vi "Delta_RH_Auto_T-waiting_simple.vi"() -> ()   [LabVIEW 2012]
uses:
  <vilib>/ptbypt/NI_PtbyPt.lvlib
panel:
  in  "T-ramp off":bool
  in  "Set He3 Temp 2":bool
  in  "Main sorb T control":bool
  in  "Wait [min]":i32
  in  "1:Main   2:Mini":dbl=1.0
  in  "LakeShore335":refnum<visa-resource-name>="COM4"
  in  "Set He3 Temp":bool
  in  "Set temp [K]":dbl=1.0
  in  "rate [K/min]":dbl=5.0
  out "Main-sorb[K]":dbl=11.567
  out "Mini sorb [K]":dbl=4.35
  in  "Temp control off":bool=TRUE
  out "temp [K]":dbl=10.729
  out "Waiting T-stability":bool caption="stabilizing"
  in  "Set Initial Field":bool
  in  "Field [T]":dbl
  in  "Period [s]":dbl=0.5 caption="Delay Time (s)"
  in  "Measure R-T":bool
  in  "Save R-T":bool
  out "R-T":cluster{"X":dbl[], "Y":dbl[]}[](graph) caption="XY Graph"
  out "Rate [K/min]":dbl=0.0015950964745404326 format="%#_6f"
  in  "Reset":bool
  in  "Stop":bool
  in  "Pause off":bool
  in  "Compliance [V]":dbl=0.5 format="%#_6f"
  out "R-H":cluster{"X":dbl[], "Y":dbl[]}[](graph)=[{"X"=[0.00063, 0.00151, 0.00233, 0.003, 0.00367, 0.00427], "Y"=[11.5344858, 11.4030008, 11.9276791, 11.5452003, 11.5064993, 11.6247473]}] caption="XY Graph"
  in  "Reset":bool
  in  "Folder":path=path "C:/User Data/Angelo/Cr-doped_NbS2/Device_Nov_2018" caption="Filename"
  out "Filename Out":path=path "C:/User Data/Angelo/Cr-doped_NbS2/Device_Nov_2018/RH-junction5-1uA_0.30K"
  in  "File name":string="RH-junction5-1uA"
  out "VTI [K]":dbl=2.07338
  out "VTI [K]":dbl=2.07412
  out "Sample Temp [K]":dbl=0.70413
  out "Magnetic Field [T]":dbl=0.00483
  out "Delta reading [Ohm]":dbl=11.5541515
  out "Delta Reading [Ohm]":dbl=11.9426813
  out "Sample Temp [K]":dbl=0.70382
  in  "Abort Delta":bool
  in  "Arm Delta":bool
  in  "DELAY [sec]":dbl=0.002 format="%#_6e"
  in  "I-HIGH [A]":dbl=1e-06 format="%#_6e"
  in  "Measure R-H":bool
  in  "Rate [K/min]":dbl=0.5
  in  "Set Temp [K]":dbl=1.0
  in  "Set Temperature":bool
  out "Magnetic Field [T]":dbl
  in  "Rate [T/min]":dbl=0.1
  in  "Set Field [T]":dbl=-0.6
  in  "Set Field":bool
  in  "Keithley":refnum<visa-resource-name>="GPIB0::20::INSTR"
  in  "Skip":bool
  in  "Wait T-stable [min]":i32=20
  in  "period (s)":dbl=0.5 min=0.0 max=1111.0 step=0.1
  in  "stop 2":bool caption="Pause"
  in  "Wait field stable [sec]":dbl=20.0
  in  "Magnet Power supply":refnum<visa-resource-name>="COM6"
  in  "Set Field [T]   Rate [T/min]":dbl[][](array[numeric])=[[0.1, 0.04], [0.6, 0.1], [0.1, 0.1], [0.0, 0.04]]
  in  "Set Temp [K]  Rate [K/min]":dbl[][](array[numeric])=[[0.3, 0.2]]
  in  "LakeShore350":refnum<visa-resource-name>="COM5"
  out "error out 3":errorcluster={"status"=FALSE, "code"=1073676294, "source"="VISA Read in Delta_RH_Auto_T-waiting_simple.vi"}
  out "error out 2":errorcluster={"status"=TRUE, "code"=-1073807339, "source"="VISA Read in Delta_RH_Auto_T-waiting_simple.vi"}
  out "error out":errorcluster={"status"=FALSE, "code"=1073676294, "source"="VISA Read in Delta_RH_Auto_T-waiting_simple.vi"}
  # "Manual control"
  # "R-H Auto Measurement"
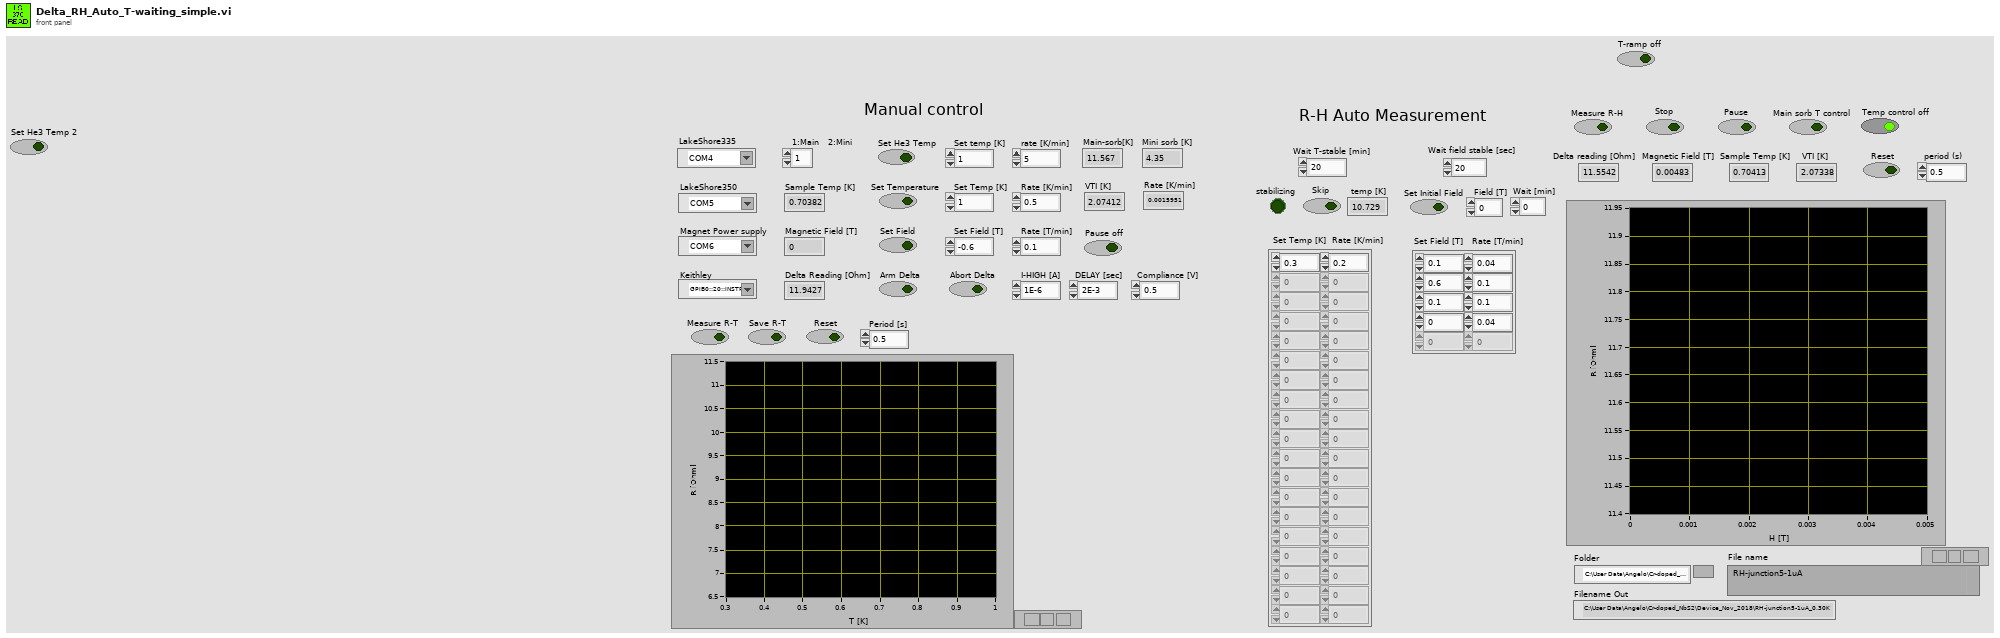
[diagram p1: front panel]
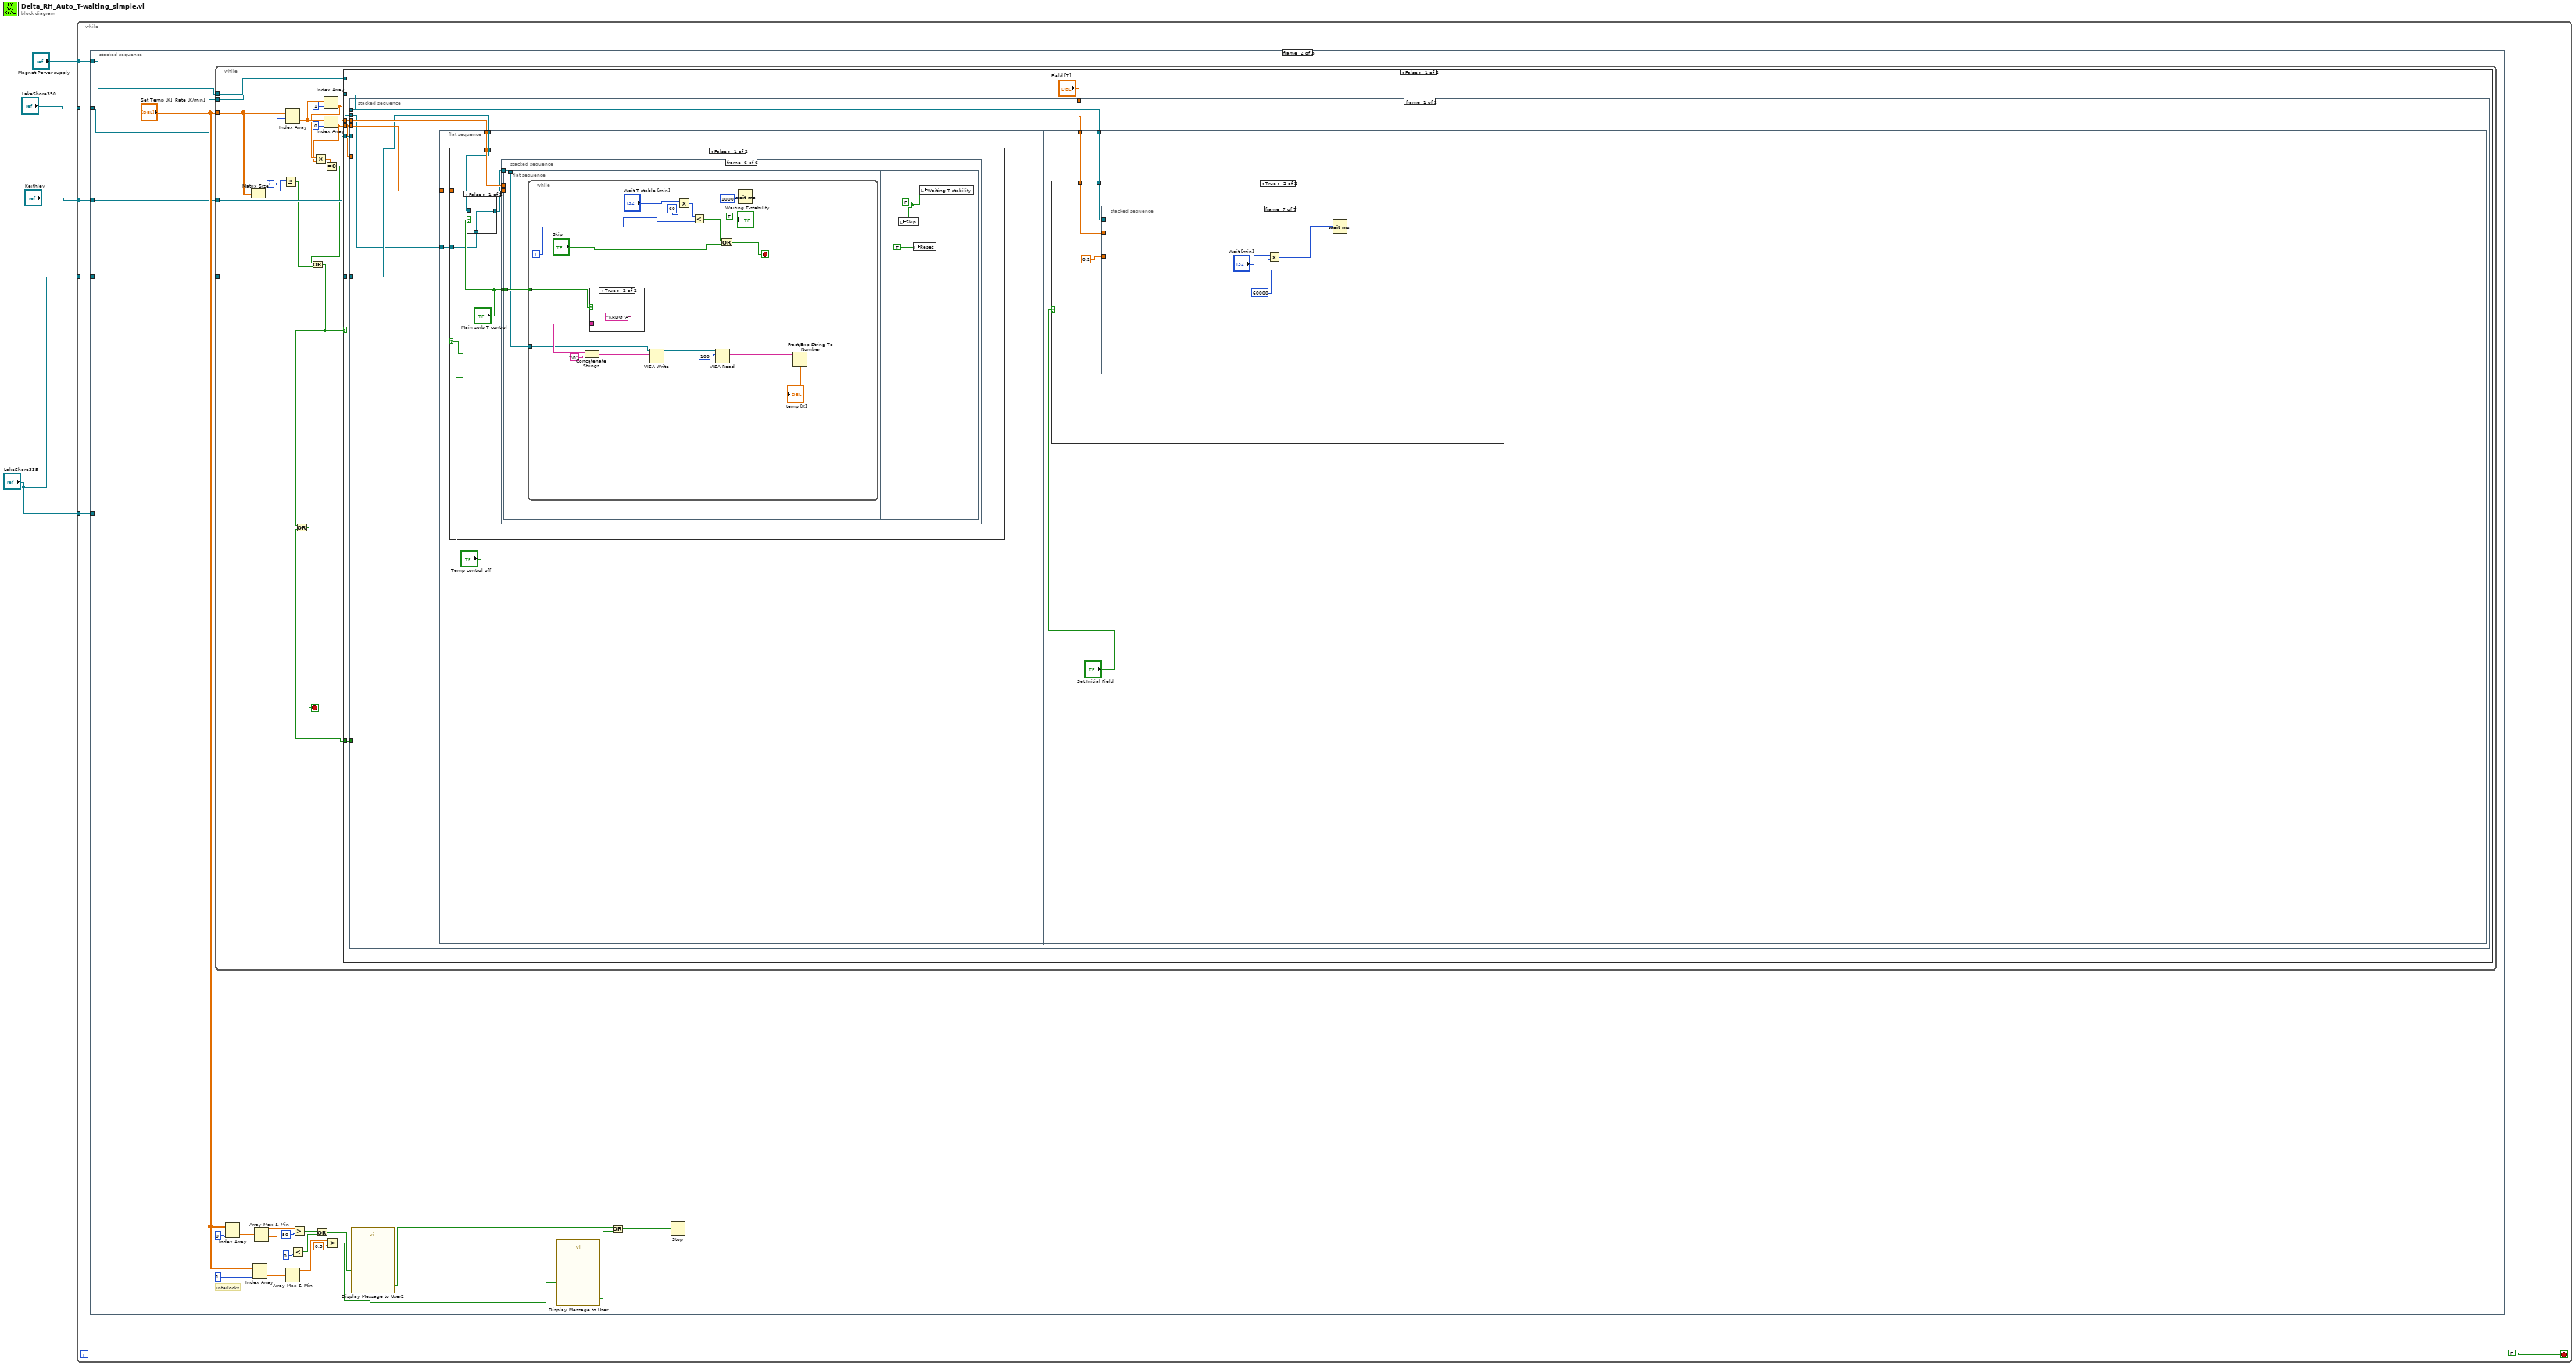
[diagram p0: block diagram]
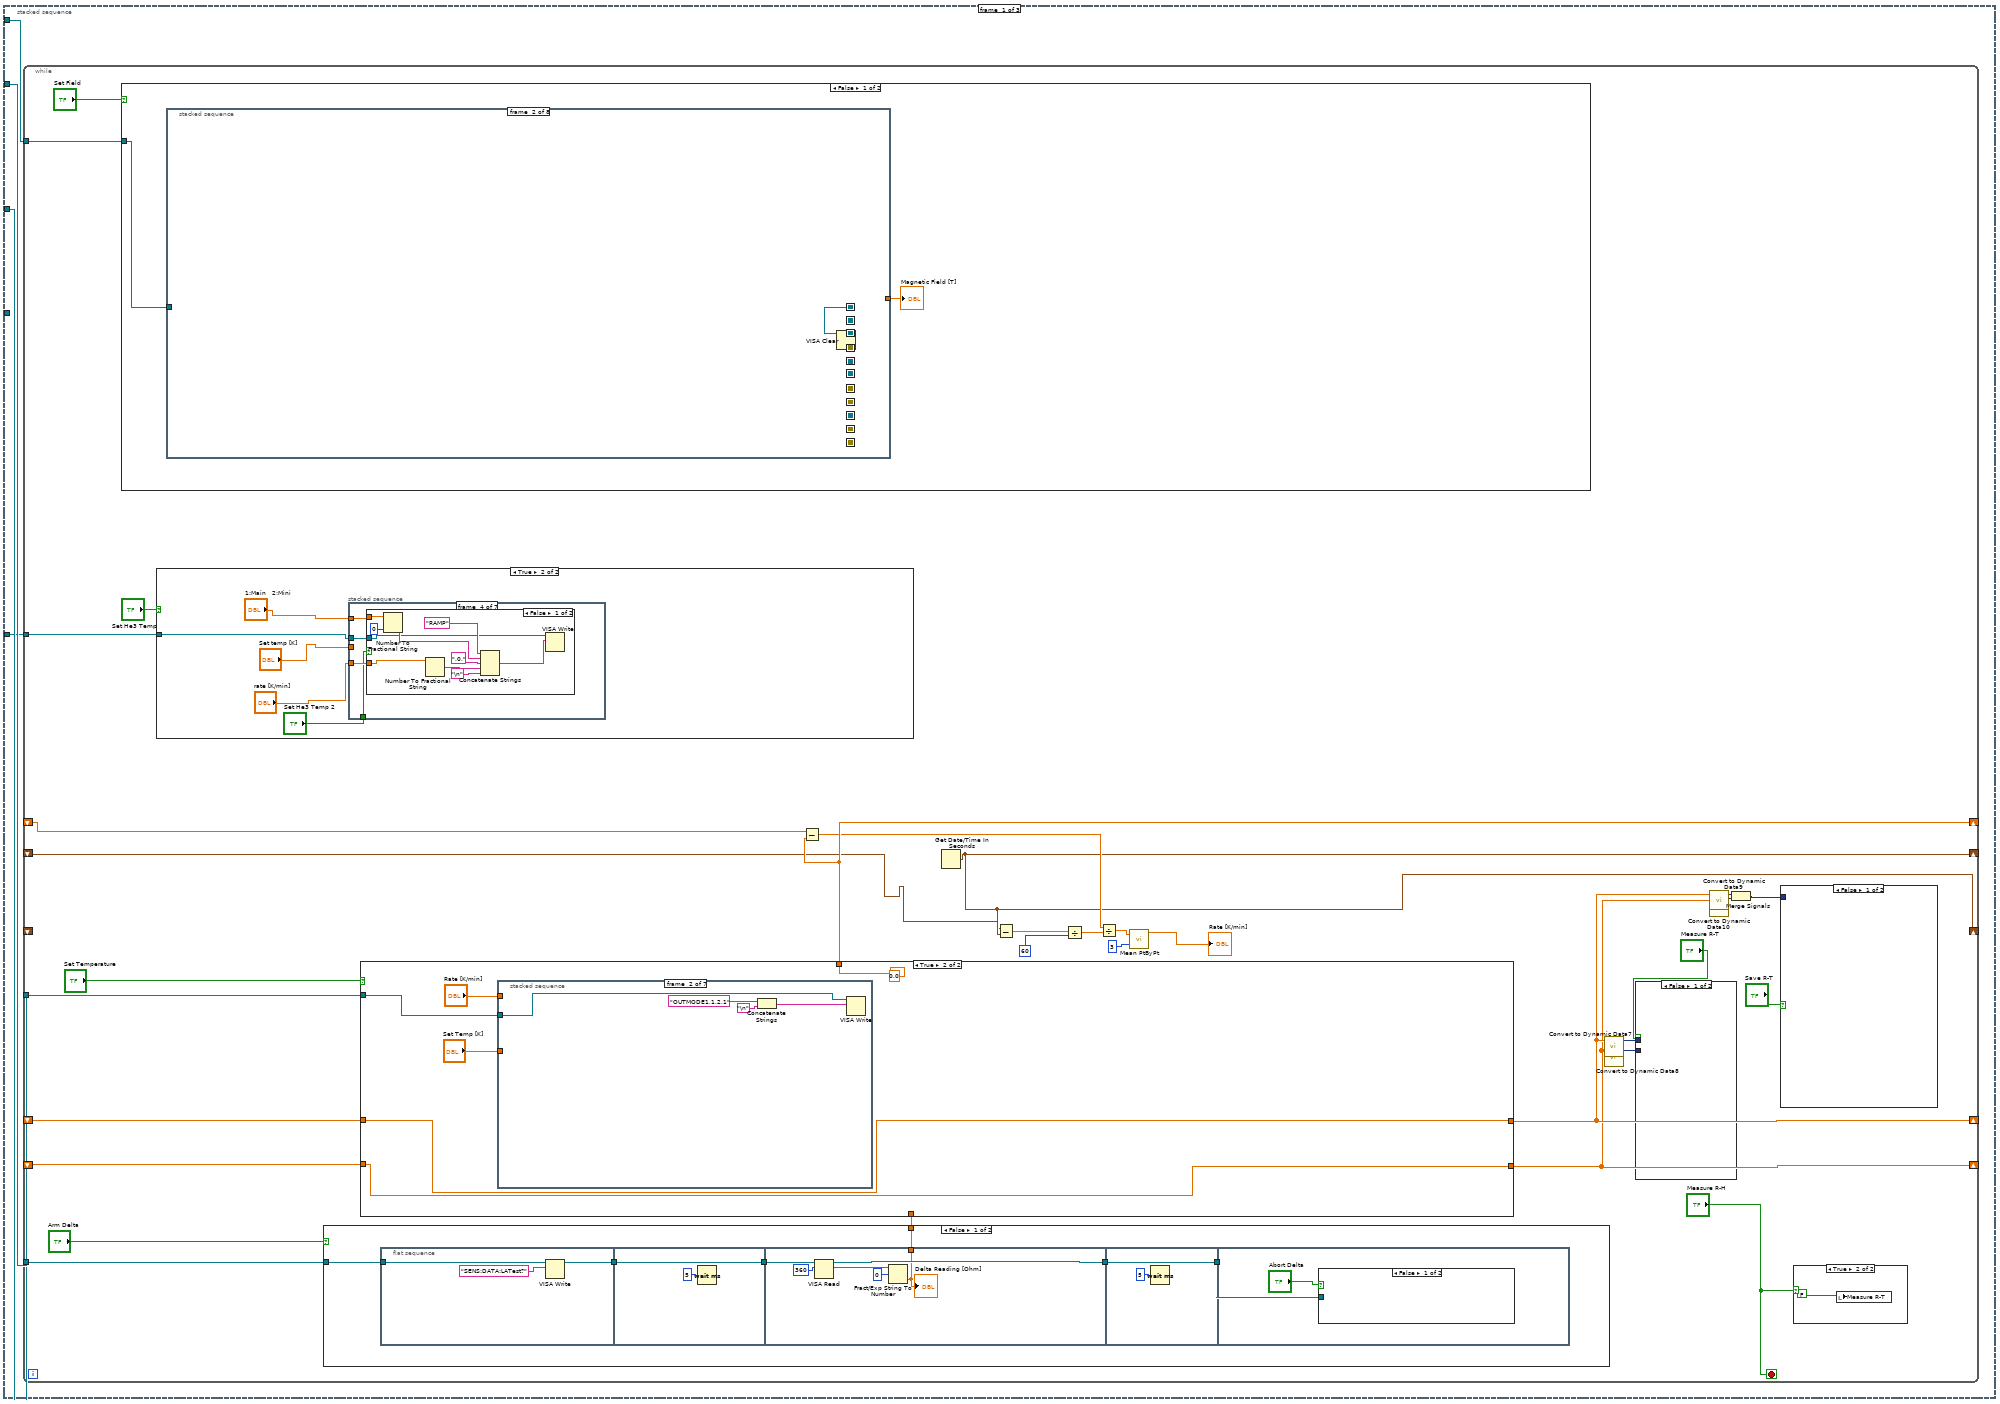
[diagram p2: hidden frame]
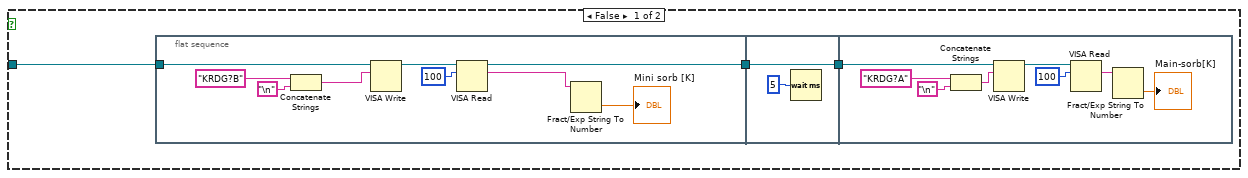
[diagram p3: hidden frame]
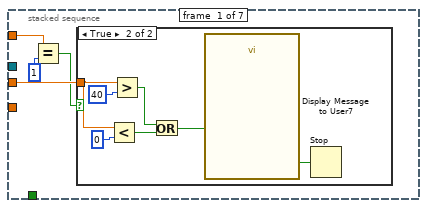
[diagram p4: hidden frame]
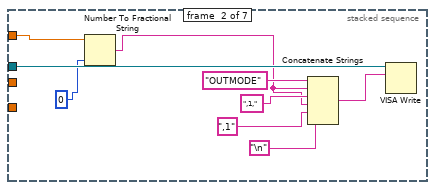
[diagram p6: hidden frame]
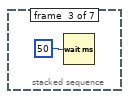
[diagram p7: hidden frame]
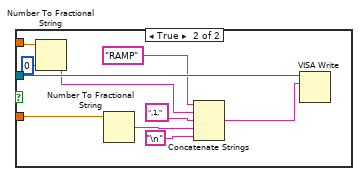
[diagram p8: hidden frame]
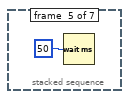
[diagram p9: hidden frame]
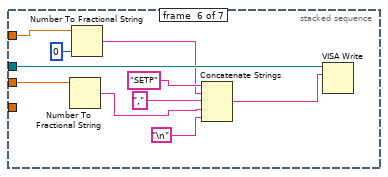
[diagram p10: hidden frame]
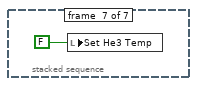
[diagram p11: hidden frame]
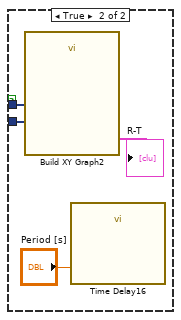
[diagram p13: hidden frame]
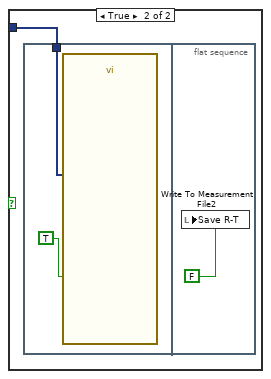
[diagram p14: hidden frame]
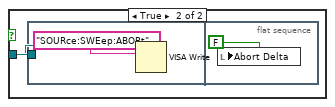
[diagram p15: hidden frame]
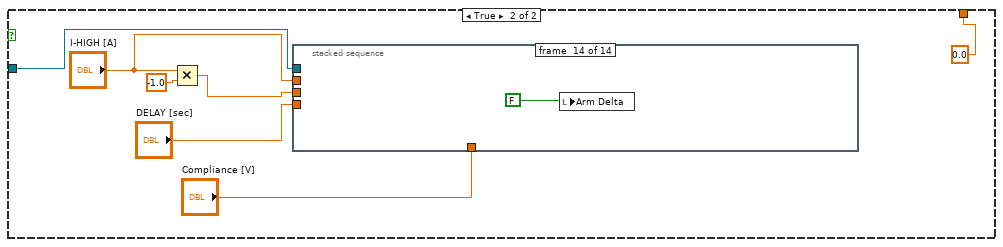
[diagram p16: hidden frame]
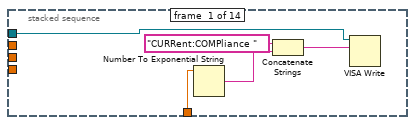
[diagram p17: hidden frame]
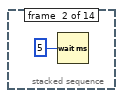
[diagram p18: hidden frame]
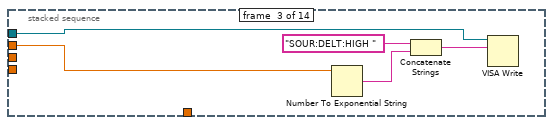
[diagram p19: hidden frame]
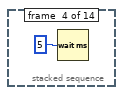
[diagram p20: hidden frame]
diagram:
  n1 = while {
    tunnel: "LakeShore350" -> [w10]
    tunnel: "Magnet Power supply" -> [w9]
    tunnel: "Keithley" -> [w8]
    tunnel: "LakeShore335" -> [w6]
    tunnel: "LakeShore335" -> [w5]
    stop <- FALSE stop-if-true
    n2 = stacked-sequence {
      tunnel: w10 -> [w13 w448 _]
      tunnel: w9 -> [w14 w447 w930]
      tunnel: w8 -> [w12 w446 _]
      tunnel: w6 -> [_ w444 _]
      tunnel: w5 -> [w11 _ _]
      frame #0 {
        n3 = while {
          tunnel: w14 -> [w41]
          tunnel: w13 -> [w44]
          tunnel: w12 -> [w43]
          shift-right: [w29] -> _
          shift-left: _ -> [w24]
          shift-right: [w27] -> _
          shift-left: _ -> [w39]
          shift-right: [w21] -> _
          shift-left: _ -> [_]
          shift-right: [w37] -> _
          shift-left: _ -> [w38]
          shift-right: [w21] -> _
          shift-left: _ -> [w20]
          tunnel: w11 -> [w15]
          stop <- "Measure R-H" stop-if-true
          n4 = case shown="False" "Set Field" {
            tunnel: w41 -> [w279 w349]
            frame False {
              n5 = stacked-sequence {
                seq-local: [w280 _ _ _ _ _ _ _] -> [_ w283 _ _ _ _ _ _]
                seq-local: [_ w281 _ _ _ _ _ _] -> [_ _ w287 _ _ _ _ _]
                seq-local: [_ w282 _ _ _ _ _ _] -> [_ _ w284 _ _ _ _ _]
                seq-local: [_ _ w286 _ _ _ _ _] -> [_ _ _ w327 _ _ _ _]
                seq-local: [_ _ w285 _ _ _ _ _] -> [_ _ _ w326 _ _ _ _]
                seq-local: [_ _ _ w329 _ _ _ _] -> [_ _ _ _ w332 _ _ _]
                seq-local: [_ _ _ w328 _ _ _ _] -> [_ _ _ _ w333 _ _ _]
                seq-local: [_ _ _ _ w332 _ _ _] -> [_ _ _ _ _ w344 _ _]
                seq-local: [_ _ _ _ w333 _ _ _] -> [_ _ _ _ _ w342 _ _]
                seq-local: [_ _ _ _ _ w343 _ _] -> [_ _ _ _ _ _ _ w348]
                seq-local: [_ _ _ _ _ w341 _ _] -> [_ _ _ _ _ _ _ w347]
                tunnel: w279 -> [w280 _ _ _ _ _ _ _]
                tunnel: [_ _ _ _ _ w334 _ _] -> w278
                frame #0 {
                }
                frame #1 {
                  n6 = VISA Clear(VISA resource name=w283) -> (VISA resource name out=w281:refnum<visa-resource-name>, error out=w282:errorcluster)  [unwired: 1 in]
                }
                frame #2 {
                  n7 = flat-sequence {
                    tunnel: w287 -> [w291]
                    tunnel: [w290] -> w286
                    tunnel: [w289] -> w285
                    tunnel: w284 -> [w288]
                    frame #0 {
                      n8 = call "Time Delay8"() -> ()  [unwired: 11 in, 1 out]
                    }
                    frame #1 {
                      n9 = case shown="False" "Pause off" {
                        tunnel: w291 -> [w294 w306]
                        tunnel: [w294 w295] -> w290
                        tunnel: [w293 w298] -> w289
                        tunnel: w288 -> [w293 w301]
                        frame False {
                        }
                        frame True {
                          n10 = flat-sequence {
                            tunnel: w306 -> [w310]
                            tunnel: [w309] -> w304
                            tunnel: [w308] -> w302
                            tunnel: w301 -> [w307]
                            tunnel: [w315] -> w305
                            tunnel: w304 -> [w315]
                            tunnel: [w314] -> w303
                            tunnel: w302 -> [w314]
                            tunnel: w305 -> [w317]
                            tunnel: w303 -> [_]
                            tunnel: [w317] -> w300
                            tunnel: [w316] -> w296
                            tunnel: w300 -> [w319]
                            tunnel: [w319] -> w299
                            tunnel: [w318] -> w297
                            tunnel: w296 -> [w318]
                            tunnel: [w323] -> w295
                            tunnel: w299 -> [w322]
                            tunnel: [w321] -> w298
                            tunnel: w297 -> [w320]
                            frame #0 {
                              n11 = Concatenate Strings("P 0" ("Command"), "\r") -> (w312:string)
                              n12 = VISA Write(VISA resource name=w310, write buffer=w312, error in (no error)=w307) -> (VISA resource name out=w309:refnum<visa-resource-name>, error out=w308:errorcluster)  [unwired: 1 out]
                            }
                            frame #1 {
                              n13 = call "Time Delay14"() -> ()  [unwired: 11 in, 1 out]
                            }
                            frame #2 {
                              n14 = VISA Close(VISA resource name=w317) -> (error out=w316:errorcluster)  [unwired: 1 in]
                            }
                            frame #3 {
                              n15 = call "Time Delay15"() -> ()  [unwired: 11 in, 1 out]
                            }
                            frame #4 {
                              n16 = VISA Clear(VISA resource name=w322, error in (no error)=w320) -> (VISA resource name out=w323:refnum<visa-resource-name>, error out=w321:errorcluster)
                            }
                            frame #5 {
                              n17 = local write "Pause off"(FALSE) -> ()
                            }
                          }
                        }
                      }
                    }
                  }
                }
                frame #3 {
                  n18 = Concatenate Strings("G O" ("Command"), "\r") -> (w330:string)
                  n19 = VISA Write(VISA resource name=w327, write buffer=w330, error in (no error)=w326) -> (VISA resource name out=w329:refnum<visa-resource-name>, error out=w328:errorcluster)  [unwired: 1 out]
                }
                frame #4 {
                  n20 = call "Time Delay9"() -> ()  [unwired: 11 in, 1 out]
                }
                frame #5 {
                  n21 = VISA Read(VISA resource name=w344, byte count=u32 30, error in (no error)=w342) -> (VISA resource name out=w343:refnum<visa-resource-name>, read buffer=w338:string, error out=w341:errorcluster)  [unwired: 1 out]
                  n22 = Match Pattern(string=w338, regular expression="OUTPUT:") -> (after substring=w336:string)  [unwired: 1 in, 3 out]
                  n23 = Match Pattern(string=w336, regular expression=" TESLA") -> (before substring=w335:string)  [unwired: 1 in, 3 out]
                  n24 = Fract/Exp String To Number(string=w335, offset=0) -> (number=w334:dbl)  [unwired: 2 in, 1 out]
                }
                frame #6 {
                  n25 = call "Time Delay10"() -> ()  [unwired: 11 in, 1 out]
                }
                frame #7 {
                  n26 = VISA Close(VISA resource name=w348, error in (no error)=w347) -> (error out=→"error out":errorcluster)
                }
              }
              "Magnetic Field [T]" <- w278
            }
            frame True {
              n27 = stacked-sequence {
                tunnel: w349 -> [w352 _ _ w371 _ w416 _ w434 _ w439 _]
                tunnel: "Set Field [T]" -> [_ w354 _ _ _ _ _ _ _ _ _]
                tunnel: "Rate [T/min]" -> [_ w353 _ _ _ _ _ w424 _ _ _]
                tunnel: "Set Field [T]" -> [_ _ _ w370 _ w414 _ _ _ _ _]
                frame #0 {
                  n28 = VISA Clear(VISA resource name=w352) -> ()  [unwired: 1 in, 2 out]
                }
                frame #1 {
                  n29 = Greater?(x=w354, y=1) -> (0:w355:bool)
                  n30 = Less?(x=w354, y=-1) -> (x < y?=w360:bool)
                  n31 = Greater?(x=w353, y=0.2) -> (0:w364:bool)
                  n32 = Less?(x=w353, y=-0.2) -> (x < y?=w363:bool)
                  n33 = Or(x=w355, y=w360) -> (x .or. y?=w366:bool)
                  n34 = Or(x=w364, y=w363) -> (x .or. y?=w365:bool)
                  n35 = call "Display Message to User6"("Enable"=w366) -> ("OK"=w367:bool)  [unwired: 9 in, 1 out]
                  n36 = call "Display Message to User5"("Enable"=w365) -> ("OK"=w356:bool)  [unwired: 9 in, 1 out]
                  n37 = Or(x=w367, y=w356) -> (x .or. y?=w357:bool)
                  n38 = Stop(stop? (T)=w357) -> ()
                }
                frame #2 {
                  n39 = Wait (ms)(milliseconds to wait=500) -> ()  [unwired: 1 out]
                }
                frame #3 {
                  # "Read Magnetic Field"
                  # "for safety"
                  # "polarity"
                  n40 = stacked-sequence {
                    seq-local: [w375 _ _ _ _ _ _ _] -> [_ w378 _ _ _ _ _ _]
                    seq-local: [_ w376 _ _ _ _ _ _] -> [_ _ w380 _ _ _ _ _]
                    seq-local: [_ w377 _ _ _ _ _ _] -> [_ _ w379 _ _ _ _ _]
                    seq-local: [_ _ w380 _ _ _ _ _] -> [_ _ _ w383 _ _ _ _]
                    seq-local: [_ _ w379 _ _ _ _ _] -> [_ _ _ w382 _ _ _ _]
                    seq-local: [_ _ _ w385 _ _ _ _] -> [_ _ _ _ w388 _ _ _]
                    seq-local: [_ _ _ w384 _ _ _ _] -> [_ _ _ _ w389 _ _ _]
                    seq-local: [_ _ _ _ w388 _ _ _] -> [_ _ _ _ _ w400 _ _]
                    seq-local: [_ _ _ _ w389 _ _ _] -> [_ _ _ _ _ w398 _ _]
                    seq-local: [_ _ _ _ _ w399 _ _] -> [_ _ _ _ _ _ _ w404]
                    seq-local: [_ _ _ _ _ w397 _ _] -> [_ _ _ _ _ _ _ w403]
                    tunnel: w371 -> [w375 _ _ _ _ _ _ _]
                    tunnel: [_ _ _ _ _ w390 _ _] -> w372
                    frame #0 {
                    }
                    frame #1 {
                      n41 = VISA Clear(VISA resource name=w378) -> (VISA resource name out=w376:refnum<visa-resource-name>, error out=w377:errorcluster)  [unwired: 1 in]
                    }
                    frame #2 {
                      n42 = call "Time Delay6"() -> ()  [unwired: 11 in, 1 out]
                    }
                    frame #3 {
                      n43 = Concatenate Strings("G O" ("Command"), "\r") -> (w386:string)
                      n44 = VISA Write(VISA resource name=w383, write buffer=w386, error in (no error)=w382) -> (VISA resource name out=w385:refnum<visa-resource-name>, error out=w384:errorcluster)  [unwired: 1 out]
                    }
                    frame #4 {
                      n45 = call "Time Delay7"() -> ()  [unwired: 11 in, 1 out]
                    }
                    frame #5 {
                      n46 = VISA Read(VISA resource name=w400, byte count=u32 30, error in (no error)=w398) -> (VISA resource name out=w399:refnum<visa-resource-name>, read buffer=w394:string, error out=w397:errorcluster)  [unwired: 1 out]
                      n47 = Match Pattern(string=w394, regular expression="OUTPUT:") -> (after substring=w392:string)  [unwired: 1 in, 3 out]
                      n48 = Match Pattern(string=w392, regular expression=" TESLA") -> (before substring=w391:string)  [unwired: 1 in, 3 out]
                      n49 = Fract/Exp String To Number(string=w391, offset=0) -> (number=w390:dbl)  [unwired: 2 in, 1 out]
                    }
                    frame #6 {
                      n50 = call "Time Delay11"() -> ()  [unwired: 11 in, 1 out]
                    }
                    frame #7 {
                      n51 = VISA Close(VISA resource name=w404, error in (no error)=w403) -> (error out=→"error out 2":errorcluster)
                    }
                  }
                  n52 = Absolute Value(x=w372) -> (abs(x)=w373:dbl)
                  n53 = Less?(x=w373, y=0.002) -> (x < y?=w369:bool)
                  n54 = case shown="True" w369 {
                    tunnel: w371 -> [_ w407]
                    tunnel: w370 -> [_ w405]
                    frame False {
                    }
                    frame True {
                      n55 = Greater Or Equal To 0?(x=w405) -> (x >= 0?=w406:bool)
                      n56 = case shown="True" w406 {
                        tunnel: ["D [-]" ("data") "D [+]" ("data")] -> w408
                        frame False {
                        }
                        frame True {
                        }
                      }
                      n57 = Concatenate Strings(w408, "\r") -> (w410:string)
                      n58 = VISA Write(VISA resource name=w407, write buffer=w410) -> ()  [unwired: 1 in, 3 out]
                    }
                  }
                }
                frame #4 {
                  n59 = Wait (ms)(milliseconds to wait=500) -> ()  [unwired: 1 out]
                }
                frame #5 {
                  # "set set field"
                  n60 = Number To Fractional String(number=w414, width (-)=i16 6, precision (6)=i16 3) -> (F-format string=w419:string)  [unwired: 1 in]
                  n61 = Concatenate Strings("S [%][MID] " ("string"), w419) -> (w415:string)
                  n62 = Concatenate Strings(w415, "\r") -> (w418:string)
                  n63 = VISA Write(VISA resource name=w416, write buffer=w418) -> ()  [unwired: 1 in, 3 out]
                }
                frame #6 {
                  n64 = Wait (ms)(milliseconds to wait=500) -> ()  [unwired: 1 out]
                }
                frame #7 {
                  # "set rate"
                  n65 = Divide(x=w424, y=60.0) -> (x/y=w429:dbl)
                  n66 = Divide(x=w429, y=0.018663) -> (x/y=w427:dbl)
                  n67 = Number To Fractional String(number=w427, width (-)=i16 6, precision (6)=i16 3) -> (F-format string=w432:string)  [unwired: 1 in]
                  n68 = Concatenate Strings("S R " ("string"), w432) -> (w431:string)
                  n69 = Concatenate Strings(w431, "\r") -> (w436:string)
                  n70 = VISA Write(VISA resource name=w434, write buffer=w436) -> ()  [unwired: 1 in, 3 out]
                }
                frame #8 {
                  n71 = Wait (ms)(milliseconds to wait=500) -> ()  [unwired: 1 out]
                }
                frame #9 {
                  # "Go to set field"
                  n72 = Concatenate Strings("R [%][MID]" ("data"), "\r") -> (w441:string)
                  n73 = VISA Write(VISA resource name=w439, write buffer=w441) -> ()  [unwired: 1 in, 3 out]
                }
                frame #10 {
                  n74 = local write "Set Field"(FALSE) -> ()
                  n75 = Wait (ms)(milliseconds to wait=500) -> ()  [unwired: 1 out]
                }
              }
            }
          }
          n76 = case shown="True" "Set He3 Temp" {
            tunnel: w15 -> [w49 w70]
            frame False {
              n77 = flat-sequence {
                tunnel: w49 -> [w52]
                tunnel: [w51] -> w47
                tunnel: [w59] -> w48
                tunnel: w47 -> [w59]
                tunnel: w48 -> [w61]
                frame #0 {
                  n78 = Concatenate Strings("KRDG?B" ("write buffer"), "\n") -> (w57:string)
                  n79 = VISA Write(VISA resource name=w52, write buffer=w57) -> (VISA resource name out=w55:refnum<visa-resource-name>)  [unwired: 1 in, 2 out]
                  n80 = VISA Read(VISA resource name=w55, byte count=u32 100) -> (VISA resource name out=w51:refnum<visa-resource-name>, read buffer=w53:string)  [unwired: 1 in, 2 out]
                  n81 = Fract/Exp String To Number(string=w53) -> (number=→"Mini sorb [K]":dbl)  [unwired: 3 in, 1 out]
                }
                frame #1 {
                  n82 = Wait (ms)(milliseconds to wait=5) -> ()  [unwired: 1 out]
                }
                frame #2 {
                  n83 = Concatenate Strings("KRDG?A" ("write buffer"), "\n") -> (w67:string)
                  n84 = VISA Write(VISA resource name=w61, write buffer=w67) -> (VISA resource name out=w65:refnum<visa-resource-name>)  [unwired: 1 in, 2 out]
                  n85 = VISA Read(VISA resource name=w65, byte count=u32 100) -> (read buffer=w63:string)  [unwired: 1 in, 3 out]
                  n86 = Fract/Exp String To Number(string=w63) -> (number=→"Main-sorb[K]":dbl)  [unwired: 3 in, 1 out]
                }
              }
            }
            frame True {
              n87 = stacked-sequence {
                tunnel: w70 -> [_ w91 _ w98 _ w126 _]
                tunnel: "Set temp [K]" -> [w77 _ _ _ _ w125 _]
                tunnel: "rate [K/min]" -> [_ _ _ w97 _ _ _]
                tunnel: "1:Main   2:Mini" -> [w76 w87 _ w96 _ w121 _]
                tunnel: "Set He3 Temp 2" -> [_ _ _ w95 _ _ _]
                frame #0 {
                  n88 = Equal?(x=w76, y=1) -> (x = y?=w74:bool)
                  n89 = case shown="True" w74 {
                    tunnel: w77 -> [_ w79]
                    frame False {
                    }
                    frame True {
                      n90 = Less?(x=w79, y=0) -> (x < y?=w83:bool)
                      n91 = Greater?(x=w79, y=40) -> (0:w80:bool)
                      n92 = Or(x=w80, y=w83) -> (x .or. y?=w84:bool)
                      n93 = call "Display Message to User7"("Enable"=w84) -> ("OK"=w78:bool)  [unwired: 9 in, 1 out]
                      n94 = Stop(stop? (T)=w78) -> ()
                    }
                  }
                }
                frame #1 {
                  n95 = Number To Fractional String(number=w87, precision (6)=i16 0) -> (F-format string=w86:string)  [unwired: 2 in]
                  n96 = Concatenate Strings("OUTMODE" ("write buffer"), w86, ",1," ("write buffer"), w86, ",1" ("write buffer"), "\n") -> (w92:string)
                  n97 = VISA Write(VISA resource name=w91, write buffer=w92) -> ()  [unwired: 1 in, 3 out]
                }
                frame #2 {
                  n98 = Wait (ms)(milliseconds to wait=u32 50) -> ()  [unwired: 1 out]
                }
                frame #3 {
                  n99 = case shown="False" w95 {
                    tunnel: w98 -> [w100 w116]
                    tunnel: w97 -> [w102 w115]
                    tunnel: w96 -> [w101 w111]
                    frame False {
                      n100 = Number To Fractional String(number=w101, precision (6)=i16 0) -> (F-format string=w103:string)  [unwired: 2 in]
                      n101 = Number To Fractional String(number=w102) -> (F-format string=w106:string)  [unwired: 3 in]
                      n102 = Concatenate Strings("RAMP" ("write buffer"), w103, ",0," ("write buffer"), w106, "\n") -> (w107:string)
                      n103 = VISA Write(VISA resource name=w100, write buffer=w107) -> ()  [unwired: 1 in, 3 out]
                    }
                    frame True {
                      n104 = Number To Fractional String(number=w111, precision (6)=i16 0) -> (F-format string=w110:string)  [unwired: 2 in]
                      n105 = Number To Fractional String(number=w115) -> (F-format string=w114:string)  [unwired: 3 in]
                      n106 = Concatenate Strings("RAMP" ("write buffer"), w110, ",1," ("write buffer"), w114, "\n") -> (w117:string)
                      n107 = VISA Write(VISA resource name=w116, write buffer=w117) -> ()  [unwired: 1 in, 3 out]
                    }
                  }
                }
                frame #4 {
                  n108 = Wait (ms)(milliseconds to wait=u32 50) -> ()  [unwired: 1 out]
                }
                frame #5 {
                  n109 = Number To Fractional String(number=w125) -> (F-format string=w124:string)  [unwired: 3 in]
                  n110 = Number To Fractional String(number=w121, precision (6)=i16 0) -> (F-format string=w122:string)  [unwired: 2 in]
                  n111 = Concatenate Strings("SETP" ("write buffer"), w122, "," ("write buffer"), w124, "\n") -> (w128:string)
                  n112 = VISA Write(VISA resource name=w126, write buffer=w128) -> ()  [unwired: 1 in, 3 out]
                }
                frame #6 {
                  n113 = local write "Set He3 Temp"(FALSE) -> ()
                }
              }
            }
          }
          n114 = case shown="False" "Arm Delta" {
            tunnel: w43 -> [w145 w169]
            tunnel: [w140 0.0] -> w40
            frame False {
              n115 = flat-sequence {
                tunnel: w145 -> [w148]
                tunnel: [w146] -> w143
                tunnel: [w149] -> w144
                tunnel: w143 -> [w149]
                tunnel: w144 -> [w153]
                tunnel: [w152] -> w141
                tunnel: [w151] -> w140
                tunnel: [w157] -> w142
                tunnel: w141 -> [w157]
                tunnel: w142 -> [w159]
                frame #0 {
                  n116 = VISA Write(VISA resource name=w148, write buffer="SENS:DATA:LATest?" ("write buffer 2")) -> (VISA resource name out=w146:refnum<visa-resource-name>)  [unwired: 1 in, 2 out]
                }
                frame #1 {
                  n117 = Wait (ms)(milliseconds to wait=5) -> ()  [unwired: 1 out]
                }
                frame #2 {
                  n118 = VISA Read(VISA resource name=w153, byte count=u32 360) -> (VISA resource name out=w152:refnum<visa-resource-name>, read buffer=w155:string)  [unwired: 1 in, 2 out]
                  n119 = Fract/Exp String To Number(string=w155, offset=0) -> (number=w151:dbl)  [unwired: 3 out]
                  "Delta Reading [Ohm]" <- w151
                }
                frame #3 {
                  n120 = Wait (ms)(milliseconds to wait=5) -> ()  [unwired: 1 out]
                }
                frame #4 {
                  n121 = case shown="False" "Abort Delta" {
                    tunnel: w159 -> [_ w161]
                    frame False {
                    }
                    frame True {
                      n122 = flat-sequence {
                        tunnel: w161 -> [w163]
                        frame #0 {
                          n123 = VISA Write(VISA resource name=w163, write buffer="SOURce:SWEep:ABORt") -> ()  [unwired: 1 in, 3 out]
                        }
                        frame #1 {
                          n124 = local write "Abort Delta"(FALSE) -> ()
                        }
                      }
                    }
                  }
                }
              }
            }
            frame True {
              n125 = Multiply(x="I-HIGH [A]", y=-1.0) -> (x*y=w168:dbl)
              n126 = stacked-sequence {
                tunnel: "I-HIGH [A]" -> [_ _ w180 _ _ _ _ _ _ _ _ _ _ _]
                tunnel: w169 -> [w173 _ w178 _ w185 _ w191 _ w196 _ w199 _ w202 _]
                tunnel: w168 -> [_ _ _ _ w184 _ _ _ _ _ _ _ _ _]
                tunnel: "DELAY [sec]" -> [_ _ _ _ _ _ w190 _ _ _ _ _ _ _]
                tunnel: "Compliance [V]" -> [w172 _ _ _ _ _ _ _ _ _ _ _ _ _]
                frame #0 {
                  n127 = Number To Exponential String(number=w172) -> (E-format string=w175:string)  [unwired: 3 in]
                  n128 = Concatenate Strings("CURRent:COMPliance ", w175) -> (w174:string)
                  n129 = VISA Write(VISA resource name=w173, write buffer=w174) -> ()  [unwired: 1 in, 3 out]
                }
                frame #1 {
                  n130 = Wait (ms)(milliseconds to wait=5) -> ()  [unwired: 1 out]
                }
                frame #2 {
                  n131 = Number To Exponential String(number=w180) -> (E-format string=w181:string)  [unwired: 3 in]
                  n132 = Concatenate Strings("SOUR:DELT:HIGH ", w181) -> (w179:string)
                  n133 = VISA Write(VISA resource name=w178, write buffer=w179) -> ()  [unwired: 1 in, 3 out]
                }
                frame #3 {
                  n134 = Wait (ms)(milliseconds to wait=5) -> ()  [unwired: 1 out]
                }
                frame #4 {
                  n135 = Number To Exponential String(number=w184) -> (E-format string=w187:string)  [unwired: 3 in]
                  n136 = Concatenate Strings("SOUR:DELT:LOW ", w187) -> (w186:string)
                  n137 = VISA Write(VISA resource name=w185, write buffer=w186) -> ()  [unwired: 1 in, 3 out]
                }
                frame #5 {
                  n138 = Wait (ms)(milliseconds to wait=5) -> ()  [unwired: 1 out]
                }
                frame #6 {
                  n139 = Number To Exponential String(number=w190) -> (E-format string=w193:string)  [unwired: 3 in]
                  n140 = Concatenate Strings("SOUR:DELT:DELay ", w193) -> (w192:string)
                  n141 = VISA Write(VISA resource name=w191, write buffer=w192) -> ()  [unwired: 1 in, 3 out]
                }
                frame #7 {
                  n142 = Wait (ms)(milliseconds to wait=5) -> ()  [unwired: 1 out]
                }
                frame #8 {
                  n143 = VISA Write(VISA resource name=w196, write buffer="UNIT OHMS ") -> ()  [unwired: 1 in, 3 out]
                }
                frame #9 {
                  n144 = Wait (ms)(milliseconds to wait=5) -> ()  [unwired: 1 out]
                }
                frame #10 {
                  n145 = VISA Write(VISA resource name=w199, write buffer="DELTa:ARM") -> ()  [unwired: 1 in, 3 out]
                }
                frame #11 {
                  n146 = Wait (ms)(milliseconds to wait=3000) -> ()  [unwired: 1 out]
                }
                frame #12 {
                  n147 = VISA Write(VISA resource name=w202, write buffer="INIT:IMM") -> ()  [unwired: 1 in, 3 out]
                }
                frame #13 {
                  n148 = local write "Arm Delta"(FALSE) -> ()
                }
              }
            }
          }
          n149 = case shown="True" "Set Temperature" {
            tunnel: w44 -> [w215 w251]
            tunnel: [w210 w248] -> w29
            tunnel: w24 -> [w211 w248]
            tunnel: w40 -> [w209 _]
            tunnel: [w208 w247] -> w27
            tunnel: w39 -> [w207 w247]
            tunnel: [w205 0.0] -> w37
            frame False {
              n150 = flat-sequence {
                tunnel: w215 -> [w229]
                tunnel: [w228] -> w213
                tunnel: [w227] -> w212
                tunnel: [w227] -> w205
                tunnel: [w236] -> w214
                tunnel: w213 -> [w236]
                tunnel: w214 -> [w238]
                frame #0 {
                  n151 = Concatenate Strings("KRDG?B" ("write buffer"), "\n") -> (w234:string)
                  n152 = VISA Write(VISA resource name=w229, write buffer=w234) -> (VISA resource name out=w232:refnum<visa-resource-name>)  [unwired: 1 in, 2 out]
                  n153 = VISA Read(VISA resource name=w232, byte count=u32 100) -> (VISA resource name out=w228:refnum<visa-resource-name>, read buffer=w230:string)  [unwired: 1 in, 2 out]
                  n154 = Fract/Exp String To Number(string=w230) -> (number=w227:dbl)  [unwired: 3 in, 1 out]
                  "Sample Temp [K]" <- w227
                }
                frame #1 {
                  n155 = Wait (ms)(milliseconds to wait=5) -> ()  [unwired: 1 out]
                }
                frame #2 {
                  n156 = Concatenate Strings("KRDG?A" ("write buffer"), "\n") -> (w244:string)
                  n157 = VISA Write(VISA resource name=w238, write buffer=w244) -> (VISA resource name out=w242:refnum<visa-resource-name>)  [unwired: 1 in, 2 out]
                  n158 = VISA Read(VISA resource name=w242, byte count=u32 100) -> (read buffer=w240:string)  [unwired: 1 in, 3 out]
                  n159 = Fract/Exp String To Number(string=w240) -> (number=→"VTI [K]":dbl)  [unwired: 3 in, 1 out]
                }
              }
              n160 = case shown="False" "Reset" {
                tunnel: w212 -> [w221 _]
                tunnel: w211 -> [w220 _]
                tunnel: [w219 w223] -> w210
                tunnel: w209 -> [w218 _]
                tunnel: [w217 w222] -> w208
                tunnel: w207 -> [w216 _]
                frame False {
                  n161 = Build Array (concatenate)(w220, w221) -> (w219:dbl[])
                  n162 = Build Array (concatenate)(w216, w218) -> (w217:dbl[])
                }
                frame True {
                  n163 = stacked-sequence {
                    tunnel: [dbl[] [] _] -> w223
                    tunnel: [dbl[] [] _] -> w222
                    frame #0 {
                    }
                    frame #1 {
                      n164 = local write "Reset"(FALSE) -> ()
                    }
                  }
                }
              }
            }
            frame True {
              n165 = stacked-sequence {
                tunnel: w251 -> [_ w259 _ w266 _ w273 _]
                tunnel: "Set Temp [K]" -> [w253 _ _ _ _ w271 _]
                tunnel: "Rate [K/min]" -> [_ _ _ w265 _ _ _]
                frame #0 {
                  n166 = Less?(x=w253, y=0) -> (x < y?=w257:bool)
                  n167 = Greater?(x=w253, y=12) -> (0:w254:bool)
                  n168 = Or(x=w254, y=w257) -> (x .or. y?=w258:bool)
                  n169 = call "Display Message to User8"("Enable"=w258) -> ("OK"=w252:bool)  [unwired: 9 in, 1 out]
                  n170 = Stop(stop? (T)=w252) -> ()
                }
                frame #1 {
                  n171 = Concatenate Strings("OUTMODE1,1,2,1" ("write buffer"), "\n") -> (w260:string)
                  n172 = VISA Write(VISA resource name=w259, write buffer=w260) -> ()  [unwired: 1 in, 3 out]
                }
                frame #2 {
                  n173 = Wait (ms)(milliseconds to wait=u32 50) -> ()  [unwired: 1 out]
                }
                frame #3 {
                  n174 = Number To Fractional String(number=w265) -> (F-format string=w264:string)  [unwired: 3 in]
                  n175 = Concatenate Strings("RAMP1,1," ("write buffer"), w264, "\n") -> (w268:string)
                  n176 = VISA Write(VISA resource name=w266, write buffer=w268) -> ()  [unwired: 1 in, 3 out]
                }
                frame #4 {
                  n177 = Wait (ms)(milliseconds to wait=u32 50) -> ()  [unwired: 1 out]
                }
                frame #5 {
                  n178 = Number To Fractional String(number=w271) -> (F-format string=w272:string)  [unwired: 3 in]
                  n179 = Concatenate Strings("SETP1," ("write buffer"), w272, "\n") -> (w275:string)
                  n180 = VISA Write(VISA resource name=w273, write buffer=w275) -> ()  [unwired: 1 in, 3 out]
                }
                frame #6 {
                  n181 = local write "Set Temperature"(FALSE) -> ()
                }
              }
            }
          }
          n182 = Subtract(x=w38, y=w37) -> (x-y=w33:dbl)
          n183 = Get Date/Time In Seconds() -> (seconds since 1Jan1904=w21:timestamp)
          n184 = Subtract(x=w20, y=w21) -> (x-y=w36:dbl)
          n185 = Divide(x=w36, y=60) -> (x/y=w34:dbl)
          n186 = Divide(x=w33, y=w34) -> (x/y=w18:dbl)
          n187 = call <vilib>:"Mean PtByPt.vi"("x"=w18, "sample length"=3) -> ("mean"=→"Rate [K/min]":dbl)  [unwired: 2 in, 1 out]
          n188 = call "Convert to Dynamic Data7"("Array"=w29) -> ("Dynamic Data Type"=w32:dynamicdata)  [unwired: 3 in]
          n189 = call "Convert to Dynamic Data8"("Array"=w27) -> ("Dynamic Data Type"=w31:dynamicdata)  [unwired: 3 in]
          n190 = case shown="False" "Measure R-T" {
            tunnel: w32 -> [_ w135]
            tunnel: w31 -> [_ w134]
            frame False {
            }
            frame True {
              n191 = call "Build XY Graph2"("Y Input"=w134, "X Input"=w135) -> ("XY Graph"=→"R-T":cluster{"X":dbl[], "Y":dbl[]}[])  [unwired: 8 in, 1 out]
              n192 = call "Time Delay16"("Delay Time (s)"="Period [s]") -> ()  [unwired: 10 in, 1 out]
            }
          }
          n193 = call "Convert to Dynamic Data9"("Array"=w29) -> ("Dynamic Data Type"=w28:dynamicdata)  [unwired: 3 in]
          n194 = call "Convert to Dynamic Data10"("Array"=w27) -> ("Dynamic Data Type"=w26:dynamicdata)  [unwired: 3 in]
          n195 = Merge Signals(w28, w26) -> (w30:dynamicdata)
          n196 = case shown="False" "Save R-T" {
            tunnel: w30 -> [_ w136]
            frame False {
            }
            frame True {
              n197 = flat-sequence {
                tunnel: w136 -> [w137]
                frame #0 {
                  n198 = call "Write To Measurement File2"("Signals"=w137, "Reset"=TRUE) -> ()  [unwired: 15 in, 3 out]
                }
                frame #1 {
                  n199 = local write "Save R-T"(FALSE) -> ()
                }
              }
            }
          }
          n200 = case shown="True" "Measure R-H" {
            frame False {
            }
            frame True {
              n201 = local write "Measure R-T"(FALSE) -> ()
            }
          }
        }
      }
      frame #1 {
        # "interlocks"
        n202 = while {
          tunnel: "Set Temp [K]  Rate [K/min]" -> [w479]
          tunnel: w448 -> [w477]
          tunnel: w447 -> [w476]
          tunnel: w446 -> [w475]
          tunnel: w444 -> [w466]
          i -> [w478]
          stop <- w467 stop-if-true
          n203 = Matrix Size(0:w479) -> (1:w480:i32)  [unwired: 1 out]
          n204 = Less Or Equal?(x=w480, y=w478) -> (x <= y?=w470:bool)
          n205 = Index Array(array=w479, index (row)=w478) -> (element=w481:dbl[])  [unwired: 1 in]
          n206 = Index Array(array=w481, index=1) -> (element=w473:dbl)
          n207 = Index Array(array=w481, index=0) -> (element=w472:dbl)
          n208 = Multiply(x=w473, y=w472) -> (x*y=w474:dbl)
          n209 = Equal To 0?(x=w474) -> (x = 0?=w471:bool)
          n210 = Or(x=w471, y=w470) -> (x .or. y?=w469:bool)
          n211 = case shown="False" w469 {
            tunnel: w477 -> [w491 _]
            tunnel: w473 -> [w490 _]
            tunnel: w476 -> [w484 _]
            tunnel: w475 -> [w489 _]
            tunnel: w472 -> [w488 _]
            tunnel: [w487 FALSE ("Boolean")] -> w468
            tunnel: w466 -> [w485 _]
            frame False {
              n212 = stacked-sequence {
                tunnel: w491 -> [w492 w605]
                tunnel: w488 -> [w497 _]
                tunnel: w490 -> [w496 _]
                tunnel: w484 -> [w495 w604]
                tunnel: w489 -> [_ w603]
                tunnel: w488 -> [_ w602]
                tunnel: [_ w601] -> w487
                tunnel: "Field [T]" -> [w494 w600]
                tunnel: w485 -> [w493 _]
                frame #0 {
                  n213 = flat-sequence {
                    tunnel: w493 -> [w502]
                    tunnel: w497 -> [w501]
                    tunnel: w496 -> [w500]
                    tunnel: w492 -> [w498]
                    tunnel: w495 -> [w564]
                    tunnel: w494 -> [w562]
                    frame #0 {
                      n214 = case shown="False" "Temp control off" {
                        tunnel: w502 -> [w505 _]
                        tunnel: w501 -> [w508 _]
                        tunnel: w500 -> [w507 _]
                        tunnel: w498 -> [w503 _]
                        frame False {
                          n215 = case shown="False" "Main sorb T control" {
                            tunnel: w505 -> [_ w510]
                            tunnel: [w509 w510] -> w504
                            tunnel: w503 -> [w509 _]
                            frame False {
                            }
                            frame True {
                            }
                          }
                          n216 = stacked-sequence {
                            tunnel: w504 -> [w511 _ w521 _ w531 w535]
                            tunnel: w508 -> [_ _ _ _ w530 _]
                            tunnel: w507 -> [_ _ w522 _ _ _]
                            tunnel: "Main sorb T control" -> [w512 _ _ _ _ w536]
                            frame #0 {
                              n217 = case shown="False" w512 {
                                tunnel: ["OUTMODE1,1,2,1" ("write buffer") "OUTMODE1,1,1,1" ("write buffer")] -> w513
                                frame False {
                                }
                                frame True {
                                }
                              }
                              n218 = Concatenate Strings(w513, "\n") -> (w514:string)
                              n219 = VISA Write(VISA resource name=w511, write buffer=w514) -> ()  [unwired: 1 in, 3 out]
                            }
                            frame #1 {
                              n220 = Wait (ms)(milliseconds to wait=u32 50) -> ()  [unwired: 1 out]
                            }
                            frame #2 {
                              n221 = case shown="True" "T-ramp off" {
                                tunnel: ["RAMP1,1," ("write buffer") "RAMP1,0," ("write buffer")] -> w520
                                frame False {
                                }
                                frame True {
                                }
                              }
                              n222 = Number To Fractional String(number=w522) -> (F-format string=w523:string)  [unwired: 3 in]
                              n223 = Concatenate Strings(w520, w523, "\n") -> (w524:string)
                              n224 = VISA Write(VISA resource name=w521, write buffer=w524) -> ()  [unwired: 1 in, 3 out]
                            }
                            frame #3 {
                              n225 = Wait (ms)(milliseconds to wait=u32 50) -> ()  [unwired: 1 out]
                            }
                            frame #4 {
                              n226 = Number To Fractional String(number=w530) -> (F-format string=w529:string)  [unwired: 3 in]
                              n227 = Concatenate Strings("SETP1," ("write buffer"), w529, "\n") -> (w533:string)
                              n228 = VISA Write(VISA resource name=w531, write buffer=w533) -> ()  [unwired: 1 in, 3 out]
                            }
                            frame #5 {
                              n229 = flat-sequence {
                                tunnel: w536 -> [w538]
                                tunnel: w535 -> [w537]
                                frame #0 {
                                n230 = while {
                                tunnel: w538 -> [w541]
                                tunnel: w537 -> [w540]
                                i -> [w539]
                                stop <- w553 stop-if-true
                                n231 = case shown="True" w541 {
                                tunnel: ["KRDG?B" ("write buffer") "KRDG?A" ("write buffer")] -> w542
                                frame False {
                                }
                                frame True {
                                }
                                }
                                n232 = Concatenate Strings(w542, "\n") -> (w547:string)
                                n233 = VISA Write(VISA resource name=w540, write buffer=w547) -> (VISA resource name out=w546:refnum<visa-resource-name>)  [unwired: 1 in, 2 out]
                                n234 = Multiply(x="Wait T-stable [min]", y=60) -> (x*y=w552:i32)
                                n235 = Less?(x=w552, y=w539) -> (x < y?=w551:bool)
                                n236 = VISA Read(VISA resource name=w546, byte count=u32 100) -> (read buffer=w544:string)  [unwired: 1 in, 3 out]
                                n237 = Or(x=w551, y="Skip") -> (x .or. y?=w553:bool)
                                n238 = Wait (ms)(milliseconds to wait=1000) -> ()  [unwired: 1 out]
                                n239 = Fract/Exp String To Number(string=w544) -> (number=→"temp [K]":dbl)  [unwired: 3 in, 1 out]
                                "Waiting T-stability" <- TRUE
                                }
                                }
                                frame #1 {
                                w559 = FALSE
                                n240 = local write "Skip"(w559) -> ()
                                n241 = local write "Reset"(TRUE) -> ()
                                n242 = local write "Waiting T-stability"(w559) -> ()
                                }
                              }
                            }
                          }
                        }
                        frame True {
                          n243 = local write "Reset"(TRUE) -> ()
                        }
                      }
                    }
                    frame #1 {
                      n244 = case shown="True" "Set Initial Field" {
                        tunnel: w564 -> [_ w567]
                        tunnel: w562 -> [_ w565]
                        frame False {
                        }
                        frame True {
                          n245 = stacked-sequence {
                            tunnel: w567 -> [w568 w571 _ w589 _ w594 _]
                            tunnel: 0.2 -> [_ _ _ w579 _ _ _]
                            tunnel: w565 -> [_ w569 _ _ _ _ _]
                            frame #0 {
                              n246 = VISA Clear(VISA resource name=w568) -> ()  [unwired: 1 in, 2 out]
                            }
                            frame #1 {
                              # "set set field"
                              n247 = Number To Fractional String(number=w569, width (-)=i16 6, precision (6)=i16 3) -> (F-format string=w574:string)  [unwired: 1 in]
                              n248 = Concatenate Strings("S [%][MID] " ("string"), w574) -> (w570:string)
                              n249 = Concatenate Strings(w570, "\r") -> (w573:string)
                              n250 = VISA Write(VISA resource name=w571, write buffer=w573) -> ()  [unwired: 1 in, 3 out]
                            }
                            frame #2 {
                              n251 = Wait (ms)(milliseconds to wait=500) -> ()  [unwired: 1 out]
                            }
                            frame #3 {
                              # "set rate"
                              n252 = Divide(x=w579, y=60.0) -> (x/y=w584:dbl)
                              n253 = Divide(x=w584, y=0.018663) -> (x/y=w582:dbl)
                              n254 = Number To Fractional String(number=w582, width (-)=i16 6, precision (6)=i16 3) -> (F-format string=w587:string)  [unwired: 1 in]
                              n255 = Concatenate Strings("S R " ("string"), w587) -> (w586:string)
                              n256 = Concatenate Strings(w586, "\r") -> (w591:string)
                              n257 = VISA Write(VISA resource name=w589, write buffer=w591) -> ()  [unwired: 1 in, 3 out]
                            }
                            frame #4 {
                              n258 = Wait (ms)(milliseconds to wait=500) -> ()  [unwired: 1 out]
                            }
                            frame #5 {
                              # "Go to set field"
                              n259 = Concatenate Strings("R [%][MID]" ("data"), "\r") -> (w596:string)
                              n260 = VISA Write(VISA resource name=w594, write buffer=w596) -> ()  [unwired: 1 in, 3 out]
                            }
                            frame #6 {
                              n261 = Multiply(x="Wait [min]", y=60000) -> (x*y=w599:i32)
                              n262 = Wait (ms)(milliseconds to wait=w599) -> ()  [unwired: 1 out]
                            }
                          }
                        }
                      }
                    }
                  }
                }
                frame #1 {
                  n263 = flat-sequence {
                    tunnel: [w621] -> w612
                    tunnel: [w622] -> w611
                    tunnel: ["Set Field [T]   Rate [T/min]"] -> w610
                    tunnel: w604 -> [w622]
                    tunnel: w603 -> [w621]
                    tunnel: w600 -> [w618]
                    tunnel: w612 -> [w646]
                    tunnel: [w646] -> w609
                    tunnel: [w645] -> w608
                    tunnel: w611 -> [w645]
                    tunnel: [w645] -> w607
                    tunnel: [w644] -> w606
                    tunnel: w610 -> [w644]
                    tunnel: w609 -> [w653]
                    tunnel: w608 -> [w652]
                    tunnel: w607 -> [w651]
                    tunnel: w606 -> [w650]
                    tunnel: w605 -> [w649]
                    tunnel: w602 -> [w648]
                    tunnel: [w647] -> w601
                    frame #0 {
                      # "interlocks"
                      n264 = Index Array(array="Set Field [T]   Rate [T/min]", index (col)=0) -> (element=w630:dbl[])  [unwired: 1 in]
                      n265 = Array Max & Min(array=w630) -> (max value=w623:dbl, min value=w633:dbl)  [unwired: 2 out]
                      n266 = Index Array(array="Set Field [T]   Rate [T/min]", index (col)=1) -> (element=w641:dbl[])  [unwired: 1 in]
                      n267 = Array Max & Min(array=w641) -> (max value=w635:dbl, min value=w638:dbl)  [unwired: 2 out]
                      n268 = Greater?(x=w623, y=1) -> (0:w624:bool)
                      n269 = Less?(x=w633, y=-1) -> (x < y?=w634:bool)
                      n270 = Greater?(x=w618, y=1) -> (0:w617:bool)
                      n271 = Less?(x=w618, y=-1) -> (x < y?=w616:bool)
                      n272 = Or(x=w624, y=w634) -> (x .or. y?=w614:bool)
                      n273 = Or(x=w617, y=w616) -> (x .or. y?=w615:bool)
                      n274 = Greater?(x=w635, y=0.2) -> (0:w640:bool)
                      n275 = Less?(x=w638, y=-0.2) -> (x < y?=w639:bool)
                      n276 = Or(x=w615, y=w614) -> (x .or. y?=w613:bool)
                      n277 = call "Display Message to User4"("Enable"=w613) -> ("OK"=w643:bool)  [unwired: 9 in, 1 out]
                      n278 = Or(x=w640, y=w639) -> (x .or. y?=w642:bool)
                      n279 = call "Display Message to User3"("Enable"=w642) -> ("OK"=w625:bool)  [unwired: 9 in, 1 out]
                      n280 = Or(x=w643, y=w625) -> (x .or. y?=w626:bool)
                      n281 = Stop(stop? (T)=w626) -> ()
                    }
                    frame #1 {
                    }
                    frame #2 {
                      n282 = while {
                        tunnel: w653 -> [w671]
                        tunnel: w652 -> [w670]
                        tunnel: w651 -> [w665]
                        tunnel: w650 -> [w662]
                        tunnel: w649 -> [w661]
                        tunnel: w648 -> [w660]
                        tunnel: [w654] -> w647
                        i -> [w666]
                        stop <- w655 stop-if-true
                        n283 = Matrix Size(0:w662) -> (1:w663:i32)  [unwired: 1 out]
                        n284 = Less Or Equal?(x=w663, y=w666) -> (x <= y?=w657:bool)
                        n285 = Index Array(array=w662, index (row)=w666) -> (element=w667:dbl[])  [unwired: 1 in]
                        n286 = Index Array(array=w667, index=1) -> (element=w659:dbl)
                        n287 = Equal To 0?(x=w659) -> (x = 0?=w658:bool)
                        n288 = Or(x=w658, y=w657) -> (x .or. y?=w656:bool)
                        n289 = Index Array(array=w667, index=0) -> (element=w664:dbl)
                        n290 = case shown="False" w656 {
                          tunnel: w671 -> [w679 _]
                          tunnel: w670 -> [w678 _]
                          tunnel: w659 -> [w677 _]
                          tunnel: w665 -> [w676 _]
                          tunnel: w664 -> [w675 _]
                          tunnel: w661 -> [w674 _]
                          tunnel: w660 -> [w673 _]
                          tunnel: [w672 FALSE] -> w654
                          frame False {
                            n291 = stacked-sequence {
                              tunnel: w679 -> [_ w763]
                              tunnel: w678 -> [_ w762]
                              tunnel: w676 -> [w682 _]
                              tunnel: w675 -> [w681 w761]
                              tunnel: w677 -> [w680 _]
                              tunnel: w674 -> [_ w760]
                              tunnel: w673 -> [_ w759]
                              tunnel: [_ w758] -> w672
                              frame #0 {
                                n292 = stacked-sequence {
                                tunnel: w681 -> [_ _ w690 _ w733 _ _ _ _ _]
                                tunnel: w682 -> [w683 _ w686 _ w730 _ w749 _ w754 _]
                                tunnel: w680 -> [_ _ _ _ _ _ w742 _ _ _]
                                frame #0 {
                                n293 = VISA Clear(VISA resource name=w683) -> ()  [unwired: 1 in, 2 out]
                                }
                                frame #1 {
                                n294 = Wait (ms)(milliseconds to wait=500) -> ()  [unwired: 1 out]
                                }
                                frame #2 {
                                # "Read Magnetic Field"
                                # "for safety"
                                # "polarity"
                                n295 = stacked-sequence {
                                seq-local: [w691 _ _ _ _ _ _ _] -> [_ w694 _ _ _ _ _ _]
                                seq-local: [_ w692 _ _ _ _ _ _] -> [_ _ w696 _ _ _ _ _]
                                seq-local: [_ w693 _ _ _ _ _ _] -> [_ _ w695 _ _ _ _ _]
                                seq-local: [_ _ w696 _ _ _ _ _] -> [_ _ _ w699 _ _ _ _]
                                seq-local: [_ _ w695 _ _ _ _ _] -> [_ _ _ w698 _ _ _ _]
                                seq-local: [_ _ _ w701 _ _ _ _] -> [_ _ _ _ w704 _ _ _]
                                seq-local: [_ _ _ w700 _ _ _ _] -> [_ _ _ _ w705 _ _ _]
                                seq-local: [_ _ _ _ w704 _ _ _] -> [_ _ _ _ _ w716 _ _]
                                seq-local: [_ _ _ _ w705 _ _ _] -> [_ _ _ _ _ w714 _ _]
                                seq-local: [_ _ _ _ _ w715 _ _] -> [_ _ _ _ _ _ _ w719]
                                seq-local: [_ _ _ _ _ w713 _ _] -> [_ _ _ _ _ _ _ w718]
                                tunnel: w686 -> [w691 _ _ _ _ _ _ _]
                                tunnel: [_ _ _ _ _ w706 _ _] -> w687
                                frame #0 {
                                }
                                frame #1 {
                                n296 = VISA Clear(VISA resource name=w694) -> (VISA resource name out=w692:refnum<visa-resource-name>, error out=w693:errorcluster)  [unwired: 1 in]
                                }
                                frame #2 {
                                n297 = call "Time Delay4"() -> ()  [unwired: 11 in, 1 out]
                                }
                                frame #3 {
                                n298 = Concatenate Strings("G O" ("Command"), "\r") -> (w702:string)
                                n299 = VISA Write(VISA resource name=w699, write buffer=w702, error in (no error)=w698) -> (VISA resource name out=w701:refnum<visa-resource-name>, error out=w700:errorcluster)  [unwired: 1 out]
                                }
                                frame #4 {
                                n300 = call "Time Delay5"() -> ()  [unwired: 11 in, 1 out]
                                }
                                frame #5 {
                                n301 = VISA Read(VISA resource name=w716, byte count=u32 30, error in (no error)=w714) -> (VISA resource name out=w715:refnum<visa-resource-name>, read buffer=w710:string, error out=w713:errorcluster)  [unwired: 1 out]
                                n302 = Match Pattern(string=w710, regular expression="OUTPUT:") -> (after substring=w708:string)  [unwired: 1 in, 3 out]
                                n303 = Match Pattern(string=w708, regular expression=" TESLA") -> (before substring=w707:string)  [unwired: 1 in, 3 out]
                                n304 = Fract/Exp String To Number(string=w707, offset=0) -> (number=w706:dbl)  [unwired: 2 in, 1 out]
                                }
                                frame #6 {
                                n305 = call "Time Delay13"() -> ()  [unwired: 11 in, 1 out]
                                }
                                frame #7 {
                                n306 = VISA Close(VISA resource name=w719, error in (no error)=w718) -> ()  [unwired: 1 out]
                                }
                                }
                                n307 = Absolute Value(x=w687) -> (abs(x)=w688:dbl)
                                n308 = Less?(x=w688, y=0.002) -> (x < y?=w685:bool)
                                n309 = case shown="False" w685 {
                                tunnel: w690 -> [_ w721]
                                tunnel: w686 -> [_ w722]
                                frame False {
                                }
                                frame True {
                                n310 = Greater Or Equal To 0?(x=w721) -> (x >= 0?=w720:bool)
                                n311 = case shown="True" w720 {
                                tunnel: ["D [-]" ("data") "D [+]" ("data")] -> w723
                                frame False {
                                }
                                frame True {
                                }
                                }
                                n312 = Concatenate Strings(w723, "\r") -> (w725:string)
                                n313 = VISA Write(VISA resource name=w722, write buffer=w725) -> ()  [unwired: 1 in, 3 out]
                                }
                                }
                                }
                                frame #3 {
                                n314 = Wait (ms)(milliseconds to wait=500) -> ()  [unwired: 1 out]
                                }
                                frame #4 {
                                # "set set field"
                                n315 = Number To Fractional String(number=w733, width (-)=i16 6, precision (6)=i16 3) -> (F-format string=w734:string)  [unwired: 1 in]
                                n316 = Concatenate Strings("S [%][MID] " ("string"), w734) -> (w729:string)
                                n317 = Concatenate Strings(w729, "\r") -> (w732:string)
                                n318 = VISA Write(VISA resource name=w730, write buffer=w732) -> ()  [unwired: 1 in, 3 out]
                                }
                                frame #5 {
                                n319 = Wait (ms)(milliseconds to wait=500) -> ()  [unwired: 1 out]
                                }
                                frame #6 {
                                # "set rate"
                                n320 = Divide(x=w742, y=60.0) -> (x/y=w744:dbl)
                                n321 = Divide(x=w744, y=0.018663) -> (x/y=w739:dbl)
                                n322 = Number To Fractional String(number=w739, width (-)=i16 6, precision (6)=i16 3) -> (F-format string=w747:string)  [unwired: 1 in]
                                n323 = Concatenate Strings("S R " ("string"), w747) -> (w746:string)
                                n324 = Concatenate Strings(w746, "\r") -> (w751:string)
                                n325 = VISA Write(VISA resource name=w749, write buffer=w751) -> ()  [unwired: 1 in, 3 out]
                                }
                                frame #7 {
                                n326 = Wait (ms)(milliseconds to wait=500) -> ()  [unwired: 1 out]
                                }
                                frame #8 {
                                # "Go to set field"
                                n327 = Concatenate Strings("R [%][MID]" ("data"), "\r") -> (w756:string)
                                n328 = VISA Write(VISA resource name=w754, write buffer=w756) -> ()  [unwired: 1 in, 3 out]
                                }
                                frame #9 {
                                n329 = Wait (ms)(milliseconds to wait=500) -> ()  [unwired: 1 out]
                                }
                                }
                              }
                              frame #1 {
                                n330 = while {
                                tunnel: w763 -> [w779]
                                tunnel: w762 -> [w780]
                                tunnel: w761 -> [w778]
                                tunnel: w760 -> [w776]
                                tunnel: w759 -> [w775]
                                shift-right: [w767] -> _
                                shift-left: _ -> [w774]
                                shift-right: [w770] -> _
                                shift-left: _ -> [w773]
                                shift-right: [w769] -> _
                                shift-left: _ -> [w772]
                                shift-right: [w768] -> _
                                shift-left: _ -> [w771]
                                tunnel: ["Stop"] -> w758
                                stop <- w766 stop-if-true
                                n331 = while {
                                stop <- "stop 2" continue-if-true
                                }
                                n332 = stacked-sequence {
                                seq-local: [w783 _ _ _ _ _] -> [_ w797 _ _ _ _]
                                seq-local: [w782 _ _ _ _ _] -> [_ w796 _ _ _ _]
                                seq-local: [_ w801 _ _ _ _] -> [_ _ w813 _ _ _]
                                seq-local: [_ w788 _ _ _ _] -> [_ _ w812 _ _ _]
                                seq-local: [_ w796 _ _ _ _] -> [_ _ w804 _ _ _]
                                seq-local: [_ w787 _ _ _ _] -> [_ _ w802 _ _ _]
                                seq-local: [_ _ w813 _ _ _] -> [_ _ _ w856 _ _]
                                seq-local: [_ _ w812 _ _ _] -> [_ _ _ w855 _ _]
                                seq-local: [_ _ w803 _ _ _] -> [_ _ _ w854 _ _]
                                seq-local: [_ _ w802 _ _ _] -> [_ _ _ w847 _ _]
                                seq-local: [_ _ _ w856 _ _] -> [_ _ _ _ w909 _]
                                seq-local: [_ _ _ w855 _ _] -> [_ _ _ _ w902 _]
                                seq-local: [_ _ _ w854 _ _] -> [_ _ _ _ w903 _]
                                seq-local: [_ _ _ w854 _ _] -> [_ _ _ _ _ _]
                                seq-local: [_ _ _ w846 _ _] -> [_ _ _ _ w899 _]
                                tunnel: w779 -> [w784 _ _ _ _ _]
                                tunnel: w780 -> [w782 _ _ _ _ _]
                                tunnel: w776 -> [_ w789 _ _ _ _]
                                tunnel: w778 -> [_ _ w811 _ _ _]
                                tunnel: [_ _ w809 _ _ _] -> w777
                                tunnel: [_ _ _ _ w909 _] -> _
                                tunnel: w775 -> [_ _ _ _ w905 _]
                                tunnel: [_ _ _ _ w885 _] -> w767
                                tunnel: w774 -> [_ _ _ _ w898 _]
                                tunnel: [_ _ _ _ w879 _] -> w770
                                tunnel: w773 -> [_ _ _ _ w892 _]
                                tunnel: [_ _ _ _ w881 _] -> w769
                                tunnel: w772 -> [_ _ _ _ w897 _]
                                tunnel: [_ _ _ _ w882 _] -> w768
                                tunnel: w771 -> [_ _ _ _ w901 _]
                                frame #0 {
                                n333 = VISA Write(VISA resource name=w784, write buffer="SENS:DATA:LATest?") -> (VISA resource name out=w783:refnum<visa-resource-name>)  [unwired: 1 in, 2 out]
                                }
                                frame #1 {
                                n334 = Concatenate Strings("KRDG?A" ("write buffer"), "\n") -> (w794:string)
                                n335 = VISA Write(VISA resource name=w789, write buffer=w794) -> (VISA resource name out=w792:refnum<visa-resource-name>)  [unwired: 1 in, 2 out]
                                n336 = VISA Read(VISA resource name=w792, byte count=u32 100) -> (VISA resource name out=w787:refnum<visa-resource-name>, read buffer=w790:string)  [unwired: 1 in, 2 out]
                                n337 = VISA Read(VISA resource name=w797, byte count=u32 360) -> (VISA resource name out=w801:refnum<visa-resource-name>, read buffer=w799:string)  [unwired: 1 in, 2 out]
                                n338 = Fract/Exp String To Number(string=w799, offset=0) -> (number=w788:dbl)  [unwired: 3 out]
                                "Delta reading [Ohm]" <- w788
                                n339 = Fract/Exp String To Number(string=w790) -> (number=→"VTI [K]":dbl)  [unwired: 3 in, 1 out]
                                }
                                frame #2 {
                                # "Read Magnetic Field"
                                n340 = stacked-sequence {
                                seq-local: [w814 _ _ _ _ _ _ _] -> [_ w817 _ _ _ _ _ _]
                                seq-local: [_ w815 _ _ _ _ _ _] -> [_ _ w819 _ _ _ _ _]
                                seq-local: [_ w816 _ _ _ _ _ _] -> [_ _ w818 _ _ _ _ _]
                                seq-local: [_ _ w819 _ _ _ _ _] -> [_ _ _ w822 _ _ _ _]
                                seq-local: [_ _ w818 _ _ _ _ _] -> [_ _ _ w821 _ _ _ _]
                                seq-local: [_ _ _ w824 _ _ _ _] -> [_ _ _ _ w827 _ _ _]
                                seq-local: [_ _ _ w823 _ _ _ _] -> [_ _ _ _ w828 _ _ _]
                                seq-local: [_ _ _ _ w827 _ _ _] -> [_ _ _ _ _ w839 _ _]
                                seq-local: [_ _ _ _ w828 _ _ _] -> [_ _ _ _ _ w837 _ _]
                                seq-local: [_ _ _ _ _ w838 _ _] -> [_ _ _ _ _ _ _ w843]
                                seq-local: [_ _ _ _ _ w836 _ _] -> [_ _ _ _ _ _ _ w842]
                                tunnel: w804 -> [w814 _ _ _ _ _ _ _]
                                tunnel: [_ _ _ _ _ w829 _ _] -> w803
                                frame #0 {
                                }
                                frame #1 {
                                n341 = VISA Clear(VISA resource name=w817) -> (VISA resource name out=w815:refnum<visa-resource-name>, error out=w816:errorcluster)  [unwired: 1 in]
                                }
                                frame #2 {
                                n342 = call "Time Delay2"() -> ()  [unwired: 11 in, 1 out]
                                }
                                frame #3 {
                                n343 = Concatenate Strings("G O" ("Command"), "\r") -> (w825:string)
                                n344 = VISA Write(VISA resource name=w822, write buffer=w825, error in (no error)=w821) -> (VISA resource name out=w824:refnum<visa-resource-name>, error out=w823:errorcluster)  [unwired: 1 out]
                                }
                                frame #4 {
                                n345 = call "Time Delay3"() -> ()  [unwired: 11 in, 1 out]
                                }
                                frame #5 {
                                n346 = VISA Read(VISA resource name=w839, byte count=u32 30, error in (no error)=w837) -> (VISA resource name out=w838:refnum<visa-resource-name>, read buffer=w833:string, error out=w836:errorcluster)  [unwired: 1 out]
                                n347 = Match Pattern(string=w833, regular expression="OUTPUT:") -> (after substring=w831:string)  [unwired: 1 in, 3 out]
                                n348 = Match Pattern(string=w831, regular expression=" TESLA") -> (before substring=w830:string)  [unwired: 1 in, 3 out]
                                n349 = Fract/Exp String To Number(string=w830, offset=0) -> (number=w829:dbl)  [unwired: 2 in, 1 out]
                                }
                                frame #6 {
                                n350 = call "Time Delay12"() -> ()  [unwired: 11 in, 1 out]
                                }
                                frame #7 {
                                n351 = VISA Close(VISA resource name=w843, error in (no error)=w842) -> (error out=→"error out 3":errorcluster)
                                }
                                }
                                "Magnetic Field [T]" <- w803
                                n352 = Equal To 0?(x=w803) -> (x = 0?=w806:bool)
                                n353 = case shown="False" w806 {
                                tunnel: w803 -> [w844 _]
                                tunnel: [w844 1.1] -> w805
                                frame False {
                                }
                                frame True {
                                }
                                }
                                n354 = Subtract(x=w805, y=w811) -> (x-y=w807:dbl)
                                n355 = Absolute Value(x=w807) -> (abs(x)=w808:dbl)
                                n356 = Less?(x=w808, y=0.001) -> (x < y?=w809:bool)
                                }
                                frame #3 {
                                n357 = Concatenate Strings("KRDG?B" ("write buffer"), "\n") -> (w852:string)
                                n358 = VISA Write(VISA resource name=w847, write buffer=w852) -> (VISA resource name out=w850:refnum<visa-resource-name>)  [unwired: 1 in, 2 out]
                                n359 = VISA Read(VISA resource name=w850, byte count=u32 100) -> (read buffer=w848:string)  [unwired: 1 in, 3 out]
                                n360 = Fract/Exp String To Number(string=w848) -> (number=w846:dbl)  [unwired: 3 in, 1 out]
                                "Sample Temp [K]" <- w846
                                }
                                frame #4 {
                                # "Temp"
                                # "Delta"
                                # "Field"
                                # "Time"
                                n361 = call "Convert to Dynamic Data5"("Array"=w892) -> ("Dynamic Data Type"=w877:dynamicdata)  [unwired: 3 in]
                                n362 = call "Convert to Dynamic Data6"("Array"=w897) -> ("Dynamic Data Type"=w876:dynamicdata)  [unwired: 3 in]
                                n363 = Number To Fractional String(number=w905, precision (6)=2) -> (F-format string=w906:string)  [unwired: 2 in]
                                n364 = call "Build XY Graph"("Y Input"=w876, "X Input"=w877) -> ("XY Graph"=→"R-H":cluster{"X":dbl[], "Y":dbl[]}[])  [unwired: 8 in, 1 out]
                                n365 = Format Date/Time String(time format string (%c)="%H:%M:%S%3u") -> (date/time string=w859:string)  [unwired: 2 in]
                                n366 = Fract/Exp String To Number(string=w859) -> (number=w860:dbl)  [unwired: 3 in, 1 out]
                                n367 = Path To String(path="Folder") -> (string=w888:string)
                                n368 = Match Pattern(string=w859, regular expression=":") -> (after substring=w865:string)  [unwired: 1 in, 3 out]
                                n369 = Fract/Exp String To Number(string=w865) -> (number=w867:dbl)  [unwired: 3 in, 1 out]
                                n370 = Match Pattern(string=w865, regular expression=":") -> (after substring=w861:string)  [unwired: 1 in, 3 out]
                                n371 = Multiply(x=w860, y=3600.0) -> (x*y=w864:dbl)
                                n372 = Concatenate Strings(w888, "\\", "File name", "_" ("string"), w906, "K") -> (w904:string)
                                n373 = Fract/Exp String To Number(string=w861) -> (number=w858:dbl)  [unwired: 3 in, 1 out]
                                n374 = Multiply(x=w867, y=60.0) -> (x*y=w863:dbl)
                                n375 = Build Array (concatenate)(w892, w903) -> (w878:dbl[])
                                n376 = Build Array (concatenate)(w897, w902) -> (w880:dbl[])
                                n377 = Build Array (concatenate)(w901, w899) -> (w883:dbl[])
                                n378 = Add(x=w864, y=w863) -> (x+y=w862:dbl)
                                n379 = Add(x=w862, y=w858) -> (x+y=w857:dbl)
                                n380 = Build Array (concatenate)(w898, w857) -> (w884:dbl[])
                                n381 = String To Path(string=w904) -> (path=w887:path)
                                n382 = call "Convert to Dynamic Data"("Array"=w884) -> ("Dynamic Data Type"=w893:dynamicdata)  [unwired: 3 in]
                                n383 = call "Convert to Dynamic Data2"("Array"=w878) -> ("Dynamic Data Type"=w896:dynamicdata)  [unwired: 3 in]
                                n384 = call "Convert to Dynamic Data4"("Array"=w883) -> ("Dynamic Data Type"=w894:dynamicdata)  [unwired: 3 in]
                                n385 = call "Convert to Dynamic Data3"("Array"=w880) -> ("Dynamic Data Type"=w895:dynamicdata)  [unwired: 3 in]
                                n386 = Merge Signals(w896, w895, w894, w893) -> (w900:dynamicdata)
                                n387 = call "Write To Measurement File"("Signals"=w900, "Reset"=TRUE, "Filename"=w887) -> ("Filename Out"=→"Filename Out":path)  [unwired: 14 in, 2 out]
                                n388 = case shown="True" "Reset" {
                                tunnel: [w913 dbl[] []] -> w885
                                tunnel: w884 -> [w913 _]
                                tunnel: w883 -> [w912 _]
                                tunnel: [w912 dbl[] []] -> w882
                                tunnel: [w911 dbl[] []] -> w881
                                tunnel: w880 -> [w911 _]
                                tunnel: [w910 dbl[] []] -> w879
                                tunnel: w878 -> [w910 _]
                                frame False {
                                }
                                frame True {
                                }
                                }
                                }
                                frame #5 {
                                n389 = local write "Reset"(FALSE) -> ()
                                }
                                }
                                n390 = call "Time Delay"("Delay Time (s)"="period (s)") -> ()  [unwired: 1 in, 10 out]
                                n391 = case shown="True" w777 {
                                tunnel: [FALSE w920] -> w765
                                frame False {
                                }
                                frame True {
                                n392 = flat-sequence {
                                tunnel: [TRUE] -> w920
                                frame #0 {
                                n393 = Multiply(x="Wait field stable [sec]", y=1000.0) -> (x*y=w921:dbl)
                                n394 = Wait (ms)(milliseconds to wait=w921) -> ()  [unwired: 1 out]
                                }
                                frame #1 {
                                }
                                }
                                }
                                }
                                n395 = Or(x="Stop", y=w765) -> (x .or. y?=w766:bool)
                                }
                              }
                            }
                          }
                          frame True {
                          }
                        }
                        n396 = Or(x=w656, y=w654) -> (x .or. y?=w655:bool)
                      }
                    }
                  }
                }
              }
            }
            frame True {
            }
          }
          n397 = Or(x=w469, y=w468) -> (x .or. y?=w467:bool)
        }
        n398 = Index Array(array="Set Temp [K]  Rate [K/min]", index (col)=0) -> (element=w456:dbl[])  [unwired: 1 in]
        n399 = Index Array(array="Set Temp [K]  Rate [K/min]", index (col)=1) -> (element=w463:dbl[])  [unwired: 1 in]
        n400 = Array Max & Min(array=w456) -> (max value=w450:dbl, min value=w459:dbl)  [unwired: 2 out]
        n401 = Array Max & Min(array=w463) -> (max value=w461:dbl)  [unwired: 3 out]
        n402 = Less?(x=w459, y=0) -> (x < y?=w460:bool)
        n403 = Greater?(x=w450, y=50) -> (0:w451:bool)
        n404 = Or(x=w451, y=w460) -> (x .or. y?=w464:bool)
        n405 = Greater?(x=w461, y=0.5) -> (0:w445:bool)
        n406 = call "Display Message to User2"("Enable"=w464) -> ("OK"=w465:bool)  [unwired: 9 in, 1 out]
        n407 = call "Display Message to User"("Enable"=w445) -> ("OK"=w452:bool)  [unwired: 9 in, 1 out]
        n408 = Or(x=w465, y=w452) -> (x .or. y?=w453:bool)
        n409 = Stop(stop? (T)=w453) -> ()
      }
      frame #2 {
        n410 = stacked-sequence {
          tunnel: w930 -> [w931 w934 _ w952 _ w957 _]
          tunnel: 0.1 -> [_ _ _ w942 _ _ _]
          tunnel: 0.0 -> [_ w932 _ _ _ _ _]
          frame #0 {
            n411 = VISA Clear(VISA resource name=w931) -> ()  [unwired: 1 in, 2 out]
          }
          frame #1 {
            # "set set field"
            n412 = Number To Fractional String(number=w932, width (-)=i16 6, precision (6)=i16 3) -> (F-format string=w937:string)  [unwired: 1 in]
            n413 = Concatenate Strings("S [%][MID] " ("string"), w937) -> (w933:string)
            n414 = Concatenate Strings(w933, "\r") -> (w936:string)
            n415 = VISA Write(VISA resource name=w934, write buffer=w936) -> ()  [unwired: 1 in, 3 out]
          }
          frame #2 {
            n416 = Wait (ms)(milliseconds to wait=500) -> ()  [unwired: 1 out]
          }
          frame #3 {
            # "set rate"
            n417 = Divide(x=w942, y=60.0) -> (x/y=w947:dbl)
            n418 = Divide(x=w947, y=0.018663) -> (x/y=w945:dbl)
            n419 = Number To Fractional String(number=w945, width (-)=i16 6, precision (6)=i16 3) -> (F-format string=w950:string)  [unwired: 1 in]
            n420 = Concatenate Strings("S R " ("string"), w950) -> (w949:string)
            n421 = Concatenate Strings(w949, "\r") -> (w954:string)
            n422 = VISA Write(VISA resource name=w952, write buffer=w954) -> ()  [unwired: 1 in, 3 out]
          }
          frame #4 {
            n423 = Wait (ms)(milliseconds to wait=500) -> ()  [unwired: 1 out]
          }
          frame #5 {
            # "Go to set field"
            n424 = Concatenate Strings("R [%][MID]" ("data"), "\r") -> (w959:string)
            n425 = VISA Write(VISA resource name=w957, write buffer=w959) -> ()  [unwired: 1 in, 3 out]
          }
          frame #6 {
            w960 = FALSE
            n426 = local write "Measure R-H"(w960) -> ()
            n427 = local write "Stop"(w960) -> ()
            n428 = Wait (ms)(milliseconds to wait=500) -> ()  [unwired: 1 out]
          }
        }
      }
    }
  }
